vi "HDF5_Write_ADAM_Record.vi"(0 "ADAM_Refs":T2 {"Group_ref" format="%.0x"; "ADAM_CoPol_dset" format="%.0x"; "ADAM_XPol_dset" format="%.0x"; "ADAM_Noise_dset" format="%.0x"; "ADAM_CalBox_dset" format="%.0x"; "TimeStamp" format="%.0x"}, 7 "HealthData":T1, 11 "error in":errorcluster) -> (15 "error out":errorcluster)   [LabVIEW 2018]
doc: "Write a single Noise<x> record with timestamp:\nNoise1\n NoiseInfo - cluster with Timestamp and other metadata for this record\n SummdSpectrum - 1024 element Double array (waveform)"
uses:
  HDF5_ADAM_Refs.ctl
  <vilib>/addons/h5labview2/base/hid_t.ctl
  HDF5_ADAM_Data.ctl
  <vilib>/addons/h5labview2/base/lib_path.vi
  <vilib>/addons/h5labview2/base/H5Equery.vi
  lib_path_mod_20200519.vi
  <vilib>/addons/h5labview2/dataset/H5Dwrite.llb/H5Dwrite.xnode
  <vilib>/addons/h5labview2/dataset/H5D.lvlib
  <vilib>/addons/h5labview2/space/H5S.lvlib
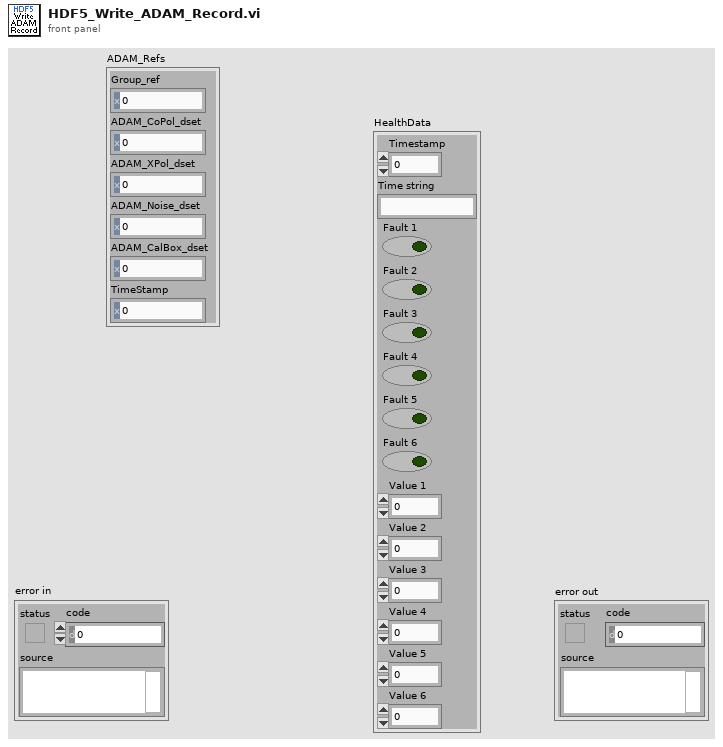
[diagram p1: front panel]
types:
  T1 = typedef "HDF5_ADAM_Data.ctl" = cluster{"Timestamp":dbl, "Time string":string, "Fault 1":bool, "Fault 2":bool, "Fault 3":bool, "Fault 4":bool, "Fault 5":bool, "Fault 6":bool, "Value 1":dbl, "Value 2":dbl, "Value 3":dbl, "Value 4":dbl, "Value 5":dbl, "Value 6":dbl}
  T2 = typedef "HDF5_ADAM_Refs.ctl" = cluster{"Group_ref":T3, "ADAM_CoPol_dset":T3, "ADAM_XPol_dset":T3, "ADAM_Noise_dset":T3, "ADAM_CalBox_dset":T3, "TimeStamp":T3}
  T3 = typedef "hid_t.ctl" = i32
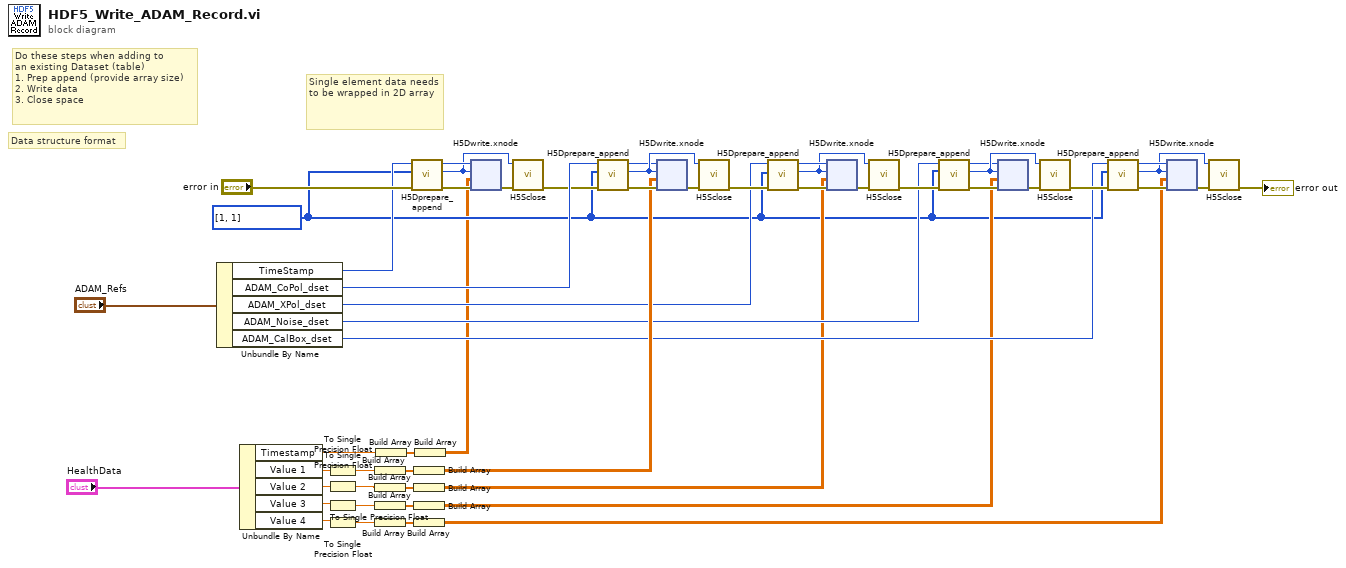
[diagram p0: block diagram]
diagram:
  w6 = u64[] [1, 1] ("append dims")
  # "Single element data needs to be wrapped in 2D array"
  # "Data structure format"
  # "Do these steps when adding to \nan existing Dataset (table)\n1. Prep append (provide array size)\n2. Write data\n3. Close space"
  n1 = Unbundle By Name("ADAM_Refs") -> ("TimeStamp"=w7:T3, "ADAM_CoPol_dset"=w20:T3, "ADAM_XPol_dset"=w19:T3, "ADAM_Noise_dset"=w18:T3, "ADAM_CalBox_dset"=w17:T3)
  n2 = Unbundle By Name("HealthData") -> ("Timestamp"=w3:dbl, "Value 1"=w47:dbl, "Value 2"=w40:dbl, "Value 3"=w41:dbl, "Value 4"=w42:dbl)
  n3 = To Single Precision Float(number=w47) -> (single precision float=w46:sgl)
  n4 = To Single Precision Float(number=w40) -> (single precision float=w39:sgl)
  n5 = To Single Precision Float(number=w41) -> (single precision float=w38:sgl)
  n6 = To Single Precision Float(number=w42) -> (single precision float=w37:sgl)
  n7 = Build Array(w46) -> (w49:sgl[])
  n8 = Build Array(w39) -> (w45:sgl[])
  n9 = Build Array(w38) -> (w44:sgl[])
  n10 = Build Array(w37) -> (w43:sgl[])
  n11 = Build Array(w3) -> (w5:dbl[])
  n12 = call <vilib>:"H5Dprepare_append.vi"("error in (no error)"="error in", "append dims"=w6, "dset in"=w7) -> ("error out"=w10:errorcluster, "space out"=w12:T3, "dset out"=w13:T3)  [unwired: 5 in, 1 out]
  n13 = Build Array(w49) -> (w48:sgl[][])
  n14 = Build Array(w45) -> (w16:sgl[][])
  n15 = Build Array(w44) -> (w15:sgl[][])
  n16 = Build Array(w43) -> (w14:sgl[][])
  n17 = Build Array(w5) -> (w4:dbl[][])
  n18 = xnode "H5Dwrite.xnode"("error in (no error)"=w10, "data"=w4, "file space"=w12, "ref in"=w13) -> ("error out"=w11:errorcluster)  [unwired: 3 in, 2 out]
  n19 = call <vilib>:"H5Sclose.vi"("error in (no error)"=w11, "space in"=w12) -> ("error out"=w9:errorcluster)  [unwired: 9 in]
  n20 = call <vilib>:"H5Dprepare_append.vi"("error in (no error)"=w9, "append dims"=w6, "dset in"=w20) -> ("error out"=w53:errorcluster, "space out"=w51:T3, "dset out"=w50:T3)  [unwired: 5 in, 1 out]
  n21 = xnode "H5Dwrite.xnode"("error in (no error)"=w53, "data"=w48, "file space"=w51, "ref in"=w50) -> ("error out"=w52:errorcluster)  [unwired: 3 in, 2 out]
  n22 = call <vilib>:"H5Sclose.vi"("error in (no error)"=w52, "space in"=w51) -> ("error out"=w24:errorcluster)  [unwired: 9 in]
  n23 = call <vilib>:"H5Dprepare_append.vi"("error in (no error)"=w24, "append dims"=w6, "dset in"=w19) -> ("error out"=w33:errorcluster, "space out"=w35:T3, "dset out"=w36:T3)  [unwired: 5 in, 1 out]
  n24 = xnode "H5Dwrite.xnode"("error in (no error)"=w33, "data"=w16, "file space"=w35, "ref in"=w36) -> ("error out"=w34:errorcluster)  [unwired: 3 in, 2 out]
  n25 = call <vilib>:"H5Sclose.vi"("error in (no error)"=w34, "space in"=w35) -> ("error out"=w23:errorcluster)  [unwired: 9 in]
  n26 = call <vilib>:"H5Dprepare_append.vi"("error in (no error)"=w23, "append dims"=w6, "dset in"=w18) -> ("error out"=w32:errorcluster, "space out"=w30:T3, "dset out"=w29:T3)  [unwired: 5 in, 1 out]
  n27 = xnode "H5Dwrite.xnode"("error in (no error)"=w32, "data"=w15, "file space"=w30, "ref in"=w29) -> ("error out"=w31:errorcluster)  [unwired: 3 in, 2 out]
  n28 = call <vilib>:"H5Sclose.vi"("error in (no error)"=w31, "space in"=w30) -> ("error out"=w22:errorcluster)  [unwired: 9 in]
  n29 = call <vilib>:"H5Dprepare_append.vi"("error in (no error)"=w22, "append dims"=w6, "dset in"=w17) -> ("error out"=w25:errorcluster, "space out"=w27:T3, "dset out"=w28:T3)  [unwired: 5 in, 1 out]
  n30 = xnode "H5Dwrite.xnode"("error in (no error)"=w25, "data"=w14, "file space"=w27, "ref in"=w28) -> ("error out"=w26:errorcluster)  [unwired: 3 in, 2 out]
  n31 = call <vilib>:"H5Sclose.vi"("error in (no error)"=w26, "space in"=w27) -> ("error out"=→"error out":errorcluster)  [unwired: 9 in]
